vi "Sample Out.vi"(8 "error in (no error)":errorcluster, 11 "Capillary Line in":refnum<class "Capillary Line.lvclass">) -> (0 "error out":errorcluster, 3 "Capillary Line out":refnum<class "Capillary Line.lvclass">)   [LabVIEW 2015, in "cRIO-Carbondioxide.lvlib" / "CO2-Actor.lvlib" / "Capillary Line.lvclass"]
uses:
  Capillary Line.lvclass
  Valve/Valve.lvclass
  Capillary Line.lvclass/Capillary Line.ctl
  CO2 Actor Messages/Ping Msg/Ping Msg.lvclass/Ping Msg.ctl
  <vilib>/ActorFramework/Message Enqueuer/Message Enqueuer.lvclass/Message Enqueuer.ctl
  <vilib>/ActorFramework/Message Enqueuer/Enqueue.vi
  <vilib>/ActorFramework/Message Priority Queue/Priority Enqueue.vi
  CO2 Actor/CO2 Actor.lvclass
  CO2 Actor Messages/Ping Msg/Ping Msg.lvclass
  <vilib>/ActorFramework/Actor/Actor.lvclass
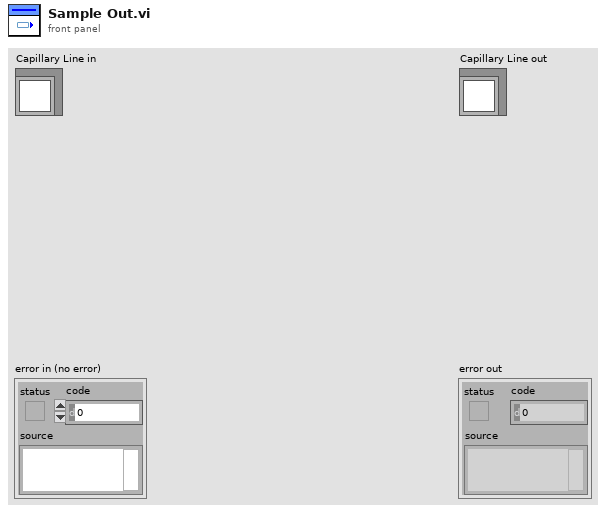
[diagram p1: front panel]
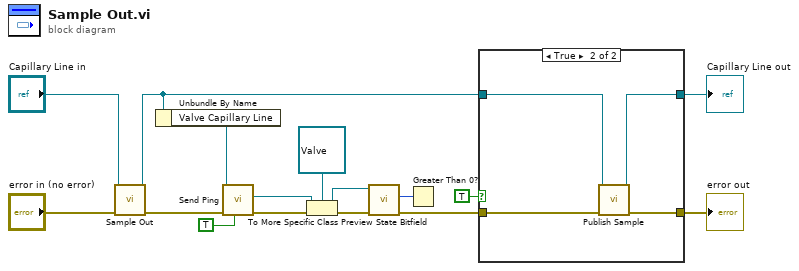
[diagram p0: block diagram]
diagram:
  n1 = call-parent "Sample Out.vi"("error in (no error)"="error in (no error)", "CO2 Actor in"="Capillary Line in") -> ("error out"=w14:errorcluster, "CO2 Actor out"=w3:refnum<class "Capillary Line.lvclass">)  [unwired: 8 in]
  n2 = Unbundle By Name(w3) -> ("Valve Capillary Line"=w13:refnum<class "Message Enqueuer.lvclass">)
  n3 = call "Send Ping.vi"("Return Self (F)"=TRUE, "error in (no error)"=w14, "Message Enqueuer"=w13) -> ("error out"=w11:errorcluster, "Actor out"=w9:refnum<class "Actor.lvclass">)  [unwired: 5 in, 2 out]
  n4 = To More Specific Class(target class=refnum<class "Valve.lvclass"> refnum ("Valve.lvclass"), reference=w9, error in=w11) -> (specific class reference=w7:refnum<class "Valve.lvclass">, error out=w8:errorcluster)
  n5 = call "Preview State Bitfield.vi"("error in (no error)"=w8, "Valve in"=w7) -> ("error out"=w4:errorcluster, "State Bitfield"=w6:u16)  [unwired: 7 in, 1 out]
  n6 = Greater Than 0?(x=w6) -> ()  [unwired: 1 out]
  n7 = case shown="True" TRUE {
    tunnel: [w17 w22] -> w5
    tunnel: w4 -> [w17 w19]
    tunnel: w3 -> [w18 w20]
    tunnel: [w18 w21] -> w2
    frame False {
    }
    frame True {
      n8 = call "Publish Sample.vi"("error in (no error)"=w19, "Capillary Line in"=w20) -> ("error out"=w22:errorcluster, "Capillary Line in 2"=w21:refnum<class "Capillary Line.lvclass">)  [unwired: 8 in]
    }
  }
  "error out" <- w5
  "Capillary Line out" <- w2
